vi "Abort Motion.vi"(8 "error in (no error)":errorcluster, 11 "FINE SIM Motion Axis":refnum<class "FINE SIM Motion Axis.lvclass">) -> (0 "error out":errorcluster, 3 "FINE SIM Motion Axis":refnum<class "FINE SIM Motion Axis.lvclass">)   [LabVIEW 2022 SP3, in "FINE SIM Motion Axis.lvclass"]
uses:
  FINE SIM Motion Axis.lvclass
  TypeDefs/Homing Status.ctl
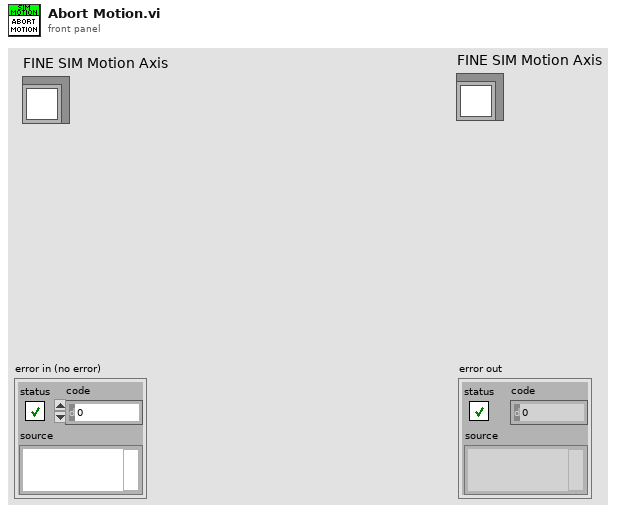
[diagram p1: front panel]
types:
  T1 = typedef "FINE SIM Motion Axis.lvclass/Homing Status.ctl" = enum16{"Idle", "Inital Home Motion", "Final Home Motion", "Done Homing"}
  T2 = typedef "FINE SIM Motion Axis.lvclass/Axis Data.ctl" = cluster{"Axis Parameters":T3, "Time Stamp":timestamp, "Settings":T4}
  T3 = typedef "FINE SIM Motion Axis.lvclass/Axis Parameters.ctl" = cluster{"Moving":bool, "Homed":bool, "Desired Position":dbl, "Current Positon":dbl, "Current Speed":dbl, "Home Status":T1}
  T4 = typedef "FINE SIM Motion Axis.lvclass/Settings.ctl" = cluster{"Axis Name":string, "Axis Settings":T5}
  T5 = typedef "FINE SIM Motion Axis.lvclass/Axis Settings.ctl" = cluster{"Speed":dbl, "Acceleration":dbl}
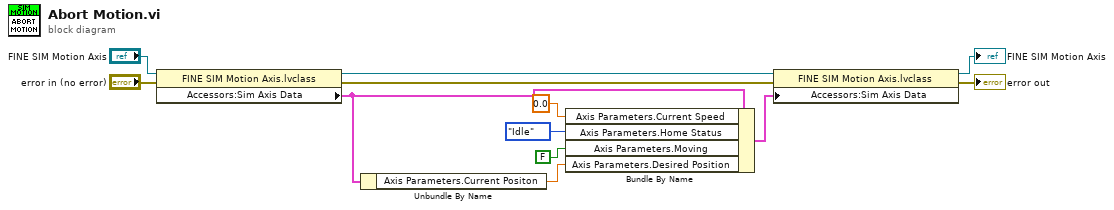
[diagram p0: block diagram]
diagram:
  n1 = property class="FINE SIM Motion Axis.lvclass"(reference="FINE SIM Motion Axis", error in="error in (no error)") -> (reference out=w12:refnum<class "FINE SIM Motion Axis.lvclass">, error out=w4:errorcluster, "Accessors:Sim Axis Data"=w11:T2)
  n2 = Unbundle By Name(w11) -> ("Axis Parameters.Current Positon"=w7:dbl)
  n3 = Bundle By Name(cluster=w11, "Axis Parameters.Current Speed"=0.0, "Axis Parameters.Home Status"=Homing_Status."Idle", "Axis Parameters.Moving"=FALSE, "Axis Parameters.Desired Position"=w7) -> (w6:T2)
  n4 = property class="FINE SIM Motion Axis.lvclass"(reference=w12, error in=w4, "Accessors:Sim Axis Data"=w6) -> (reference out=→"FINE SIM Motion Axis":refnum<class "FINE SIM Motion Axis.lvclass">, error out=→"error out":errorcluster)
